vi "配置读取.vi"(8 "error in (no error)":errorcluster) -> (0 "error out":errorcluster, 3 "配置":T1={"编码器工程变换系数_计数值"=0.0, "编码器工程变换系数_工程值"=0.0, "最小精度设置"=0.01, "剖面校正值设定"=0.0, "软限位最大值"=25.0, "软限位最小值"=2.0, "剖面待机位置设定"=0.0} {"剖面待机位置设定" format="%#_6f m"; "软限位最小值" format="%#_6f m"; "软限位最大值" format="%#_6f m"; "剖面校正值设定" format="%#_6f m"; "最小精度设置" format="%#.6f"; "编码器工程变换系数_工程值" format="%#_6f m"; "编码器工程变换系数_计数值" format="%#_6f ps"})   [LabVIEW 2016, in "PLC.lvlib"]
uses:
  PLC.lvlib
  <vilib>/Plasmionique/MB Master/MB_Master_Serial/MB_Master_Serial.lvclass
  C:/Program Files (x86)/National Instruments/LabVIEW 2016/vi.lib/Plasmionique/MB Master/MB_Master/MB_Master.lvclass
  <vilib>/Plasmionique/MB Master/MB Master.lvlib
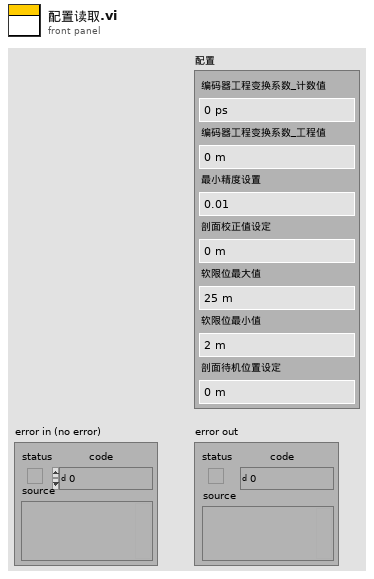
[diagram p1: front panel]
types:
  T1 = cluster{"编码器工程变换系数_计数值":sgl, "编码器工程变换系数_工程值":sgl, "最小精度设置":sgl, "剖面校正值设定":sgl, "软限位最大值":sgl, "软限位最小值":sgl, "剖面待机位置设定":sgl}
  T2 = cluster{"[0]":sgl, "[1]":sgl, "[2]":sgl, "[3]":sgl, "[4]":sgl, "[5]":sgl, "[6]":sgl}
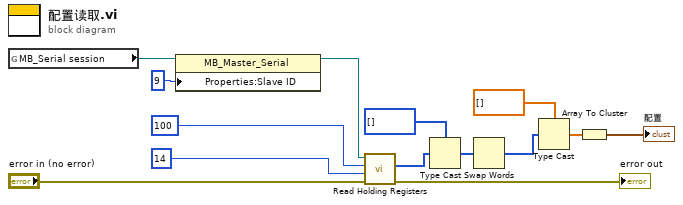
[diagram p0: block diagram]
diagram:
  n1 = global read "中间变量.vi" "MB_Serial session"() -> (w7:refnum<class "MB_Master_Serial.lvclass">)
  n2 = property class="MB_Master_Serial"(reference=w7, "Properties:Slave ID"=u8 9 ("Slave ID")) -> (reference out=w6:refnum<class "MB_Master_Serial.lvclass">)  [unwired: 1 in, 1 out]
  n3 = call <vilib>:"Read Holding Registers.vi"("error in (no error)"="error in (no error)", "quantity"=u16 14, "starting address"=u16 100, "MB session in"=w6) -> ("error out"=→"error out":errorcluster, "Registers"=w3:u16[])  [unwired: 5 in, 1 out]
  n4 = Type Cast(type=u32[] [], x=w3) -> (*(type *) &x=w10:u32[])
  n5 = Swap Words(1:w10) -> (0:w9:u32[])
  n6 = Type Cast(type=sgl[] [], x=w9) -> (*(type *) &x=w2:sgl[])
  n7 = Array To Cluster(array=w2) -> (cluster=→"配置":T2)
